vi "ConstructAuthority.vi"(8 "password":string, 9 "username":string, 10 "port":string, 11 "host":string) -> (3 "authority":string)   [LabVIEW 2013, in "openURI.lvlib"]
uses:
  openURI.lvlib
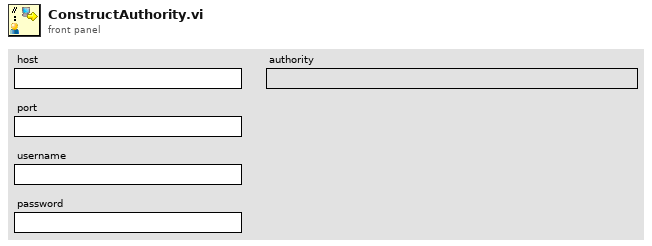
[diagram p1: front panel]
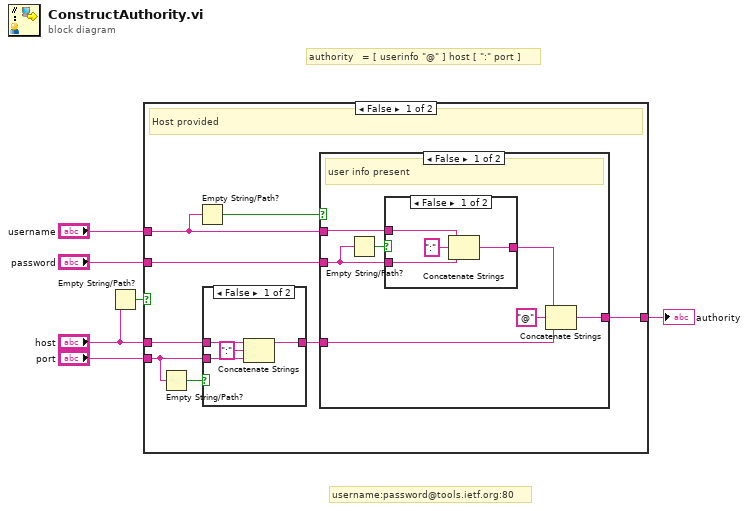
[diagram p0: block diagram]
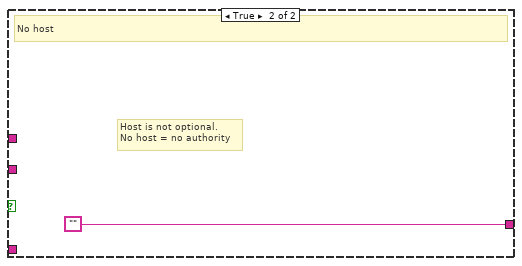
[diagram p5: hidden frame]
diagram:
  # "username:password@tools.ietf.org:80"
  # "authority   = [ userinfo \"@\" ] host [ \":\" port ]"
  n1 = Empty String/Path?(string/path="host") -> (empty?=w3:bool)
  n2 = case shown="False" w3 {
    tunnel: "username" -> [w13 _]
    tunnel: "password" -> [w12 _]
    tunnel: [w11 ""] -> w4
    tunnel: "host" -> [w8 _]
    tunnel: "port" -> [w9 _]
    frame False {
      # "Host provided"
      n3 = Empty String/Path?(string/path=w9) -> (empty?=w10:bool)
      n4 = Empty String/Path?(string/path=w13) -> (empty?=w14:bool)
      n5 = case shown="False" w10 {
        tunnel: w9 -> [w15 _]
        tunnel: [w17 w19] -> w7
        tunnel: w8 -> [w16 w19]
        frame False {
          n6 = Concatenate Strings(w16, ":" ("string"), w15) -> (w17:string)
        }
        frame True {
          # "No port"
        }
      }
      n7 = case shown="False" w14 {
        tunnel: w13 -> [w23 _]
        tunnel: w12 -> [w20 _]
        tunnel: [w25 w32] -> w11
        tunnel: w7 -> [w24 w32]
        frame False {
          # "user info present"
          n8 = Empty String/Path?(string/path=w20) -> (empty?=w21:bool)
          n9 = case shown="False" w21 {
            tunnel: w23 -> [w29 w31]
            tunnel: w20 -> [w28 _]
            tunnel: [w27 w31] -> w22
            frame False {
              n10 = Concatenate Strings(w29, ":" ("string"), w28) -> (w27:string)
            }
            frame True {
            }
          }
          n11 = Concatenate Strings(w22, "@" ("string"), w24) -> (w25:string)
        }
        frame True {
          # "No userinfo"
        }
      }
    }
    frame True {
      # "Host is not optional.\nNo host = no authority"
      # "No host"
    }
  }
  "authority" <- w4
